vi "demo.vi"() -> ()   [LabVIEW 2015]
uses:
  <vilib>/DAQmx/read.llb/DAQmx Read (Analog 1D DBL 1Chan NSamp).vi
  <vilib>/DAQmx/configure/timing.llb/DAQmx Timing (Sample Clock).vi
panel:
  out "all data":dbl[](array[numeric])
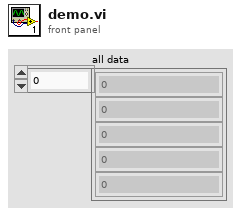
[diagram p1: front panel]
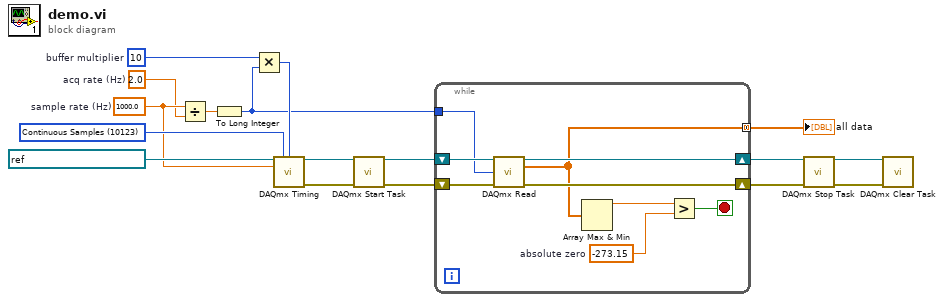
[diagram p0: block diagram]
diagram:
  w8 = 10  # buffer multiplier
  w10 = 2.0  # acq rate (Hz)
  w11 = 1000.0  # sample rate (Hz)
  w12 = 10123 items=["Finite Samples"=10178, "Continuous Samples"=10123, "Hardware Timed Single Point"=12522] ("sample mode")
  n1 = Divide(x=w11, y=w10) -> (x/y=w9:dbl)
  n2 = To Long Integer(number=w9) -> (32bit integer=w2:i32)
  n3 = Multiply(x=w8, y=w2) -> (x*y=w7:i32)
  n4 = call-poly <vilib>:"DAQmx Timing.vi"("task/channels in"=refnum<k21> "MyTemperatureTask", "sample mode"=w12, "samples per channel"=w7, "rate"=w11) -> ("task out"=w6:refnum<k21>, "error out"=w17:errorcluster)  [unwired: 10 in]
  n5 = call <vilib>:"DAQmx Start Task.vi"("task/channels in"=w6, "error in"=w17) -> ("task out"=w5:refnum<k21>, "error out"=w16:errorcluster)  [unwired: 12 in]
  n6 = while {
    shift-right: [w25] -> w15
    shift-left: w16 -> [w26]
    shift-right: [w23] -> w4
    shift-left: w5 -> [w24]
    tunnel: w2 -> [w22]
    tunnel: [w21] -> w1 mode=concatenating
    stop <- w19 stop-if-true
    w18 = -273.15  # absolute zero
    n7 = call-poly <vilib>:"DAQmx Read.vi"("task/channels in"=w24, "number of samples per channel"=w22, "error in"=w26) -> ("task out"=w23:refnum<k21>, "data"=w21:dbl[], "error out"=w25:errorcluster)  [unwired: 10 in]
    n8 = Array Max & Min(array=w21) -> (max value=w20:dbl)  [unwired: 3 out]
    n9 = Greater?(x=w20, y=w18) -> (0:w19:bool)
  }
  "all data" <- w1
  n10 = call <vilib>:"DAQmx Stop Task.vi"("task/channels in"=w4, "error in"=w15) -> ("task out"=w3:refnum<k21>, "error out"=w14:errorcluster)  [unwired: 12 in]
  n11 = call <vilib>:"DAQmx Clear Task.vi"("task in"=w3, "error in"=w14) -> ()  [unwired: 13 in, 1 out]
